vi "FromClusterToTagBus.vi"() -> ()   [LabVIEW 2013]
uses:
  Controls/SampleControl.ctl
panel:
  in  "Cluster":T1
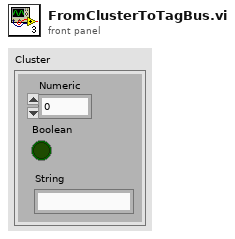
[diagram p1: front panel]
types:
  T1 = typedef "SampleControl.ctl" = cluster{"Numeric":dbl, "Boolean":bool, "String":string}
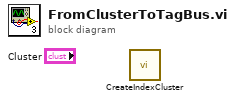
[diagram p0: block diagram]
diagram:
  n1 = call "CreateIndexCluster.vi"() -> ()  [unwired: 11 in, 1 out]
